vi "Launch Loop.vi"(8 "error in (no error)":errorcluster, 11 "Basic WebSocket Manager in":refnum<class "Basic WebSocket Manager.lvclass">) -> (0 "error out":errorcluster, 3 "Basic WebSocket Manager out":refnum<class "Basic WebSocket Manager.lvclass">)   [LabVIEW 2020, in "HTTP Server.lvlib" / "Basic WebSocket Manager.lvclass"]
uses:
  Basic WebSocket Manager.lvclass
  Basic WebSocket Manager.lvclass/Basic WebSocket Manager.ctl
  Loop Async.vi
  lv-exec-anchor/ExecAnchor/ExecAnchor.lvclass
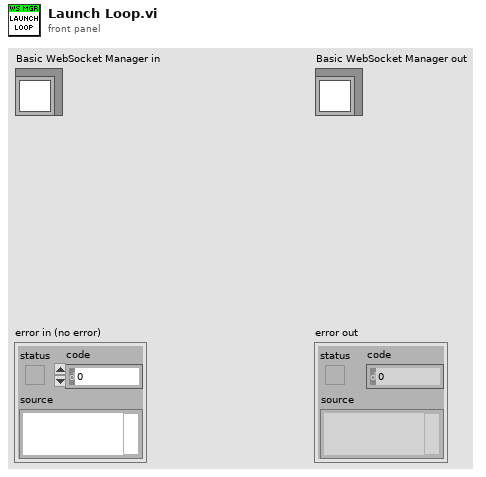
[diagram p1: front panel]
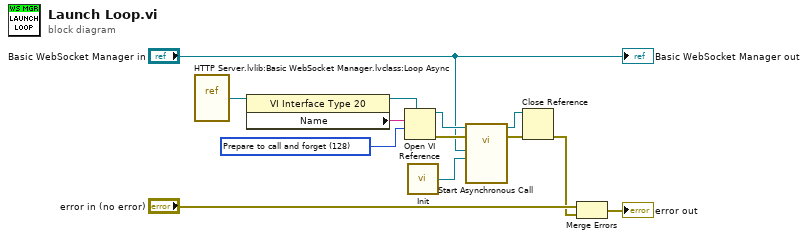
[diagram p0: block diagram]
diagram:
  w7 = 128 items=["Record modifications"=1, "Open templates for editing"=2, "Prompt user to save"=4, "Prepare for reentrant run"=8, "Prompt to find missing subVIs"=16, "Hide loading dialog box"=32, "Enable simultaneous calls"=64, "Prepare to call and forget"=128, "Simultaneous call and forget"=192, "Prepare to call and collect"=256, "Simultaneous call and collect"=320]
  n1 = vi-ref "HTTP Server.lvlib:Basic WebSocket Manager.lvclass:Loop Async.vi"() -> (w5:refnum<vi>)
  n2 = property class="VI Interface Type 20"(reference=w5) -> (reference out=w8:refnum<vi>, "Name"=w6:string)  [unwired: 1 in, 1 out]
  n3 = Open VI Reference(type specifier VI Refnum (for type only)=w8, vi path=w6, options=w7) -> (vi reference=w10:refnum<vi>, error out=w9:errorcluster)  [unwired: 3 in]
  n4 = call "Init.vi"() -> ("ExecAnchor out"=w4:refnum<class "ExecAnchor.lvclass">)  [unwired: 7 in]
  n5 = call-by-ref "Start Asynchronous Call"(reference=w10, error in=w9, "ExecAnchor"=w4, "Basic WebSocket Manager in"="Basic WebSocket Manager in") -> (reference out=w12:refnum<vi>, error out=w11:errorcluster)  [unwired: 10 in]
  n6 = Close Reference(reference=w12, error in (no error)=w11) -> (error out=w1:errorcluster)
  n7 = Merge Errors("error in (no error)", w1) -> (→"error out":errorcluster)
  "Basic WebSocket Manager out" <- "Basic WebSocket Manager in"
